vi "X-CAN_Connection_No_Stream_Connection.vi"() -> ()   [LabVIEW 2015]
uses:
  <vilib>/Stratom, Inc/X-CAN for myRIO (API)/X-CAN Class/Type Definitions/CAN_Speed.ctl
  <vilib>/Stratom, Inc/X-Modules for myRIO/Type Defs/MXPChannel.ctl
  <vilib>/Platform/TimedLoop/XDataNode/timing_clust.ctl
  <vilib>/Platform/TimedLoop/XDataNode/nitl_modes.ctl
  <vilib>/Platform/TimedLoop/XDataNode/wakeup.ctl
  <vilib>/platform/TimedLoop/XDataNode/XDataNode.xnode
  <vilib>/Stratom, Inc/X-CAN for myRIO (API)/X-CAN Class/X-CAN.lvclass
  <vilib>/Platform/TimedLoop/XDataNode/XDNodeRunTimeDep.lvlib
panel:
  out "Motor positions (degree)":T1(array[cluster]) {"Error Code (bits)" format="%b"}
  in  "Stop Button":bool
  in  "Enable Joint":bool[](array[boolean])
  in  "Reset?":bool
  in  "Desired position (degrees)":i32[](array[numeric])
  # "Base"
  # "Shoulder"
  # "Elbow"
  # "Wrist"
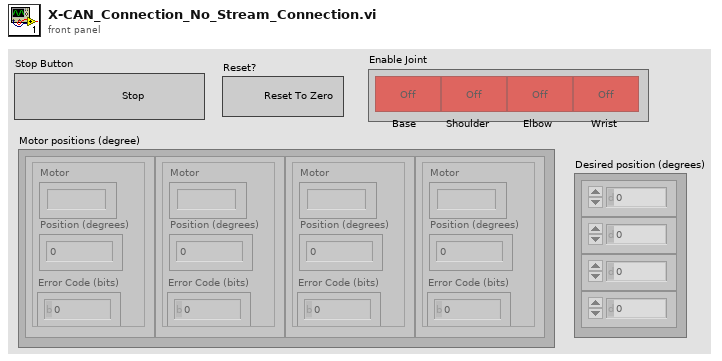
[diagram p1: front panel]
types:
  T1 = cluster{"Position (degrees)":i32, "Error Code (bits)":u8, "Motor":string}[]
  T2 = typedef "MXPChannel.ctl" = enum16{"A/MXP", "B/MXP"}
  T3 = typedef "X-CAN.lvclass/CAN_Speed.ctl" = u8
  T4 = cluster{"ID":u8, "Position":u16, "Error Code":u8}[]
  T5 = typedef "XDNodeRunTimeDep.lvlib/timing_clust.ctl" = cluster{"Expected End [f-1]":u64, "Actual End [f-1]":u64, "Finished Late? [f-1]":bool, "Expected End [i-1]":u64, "Actual End [i-1]":u64, "Finished Late? [i-1]":bool, "Expected Start [i]":u64, "Actual Start [i]":u64, "Expected Start [f]":u64, "Actual Start [f]":u64, "Source Name":string, "Structure Name":string, "Period":i64, "Deadline":i64, "Offset":i64, "Start":i64, "Priority":i32, "Timeout":i32, "Mode":T6, "Wakeup Reason":T7, "Error":errorcluster, "Source Type":string, "Secondary Source Type":string, "Global End Time":u64, "Global Start Time":u64, "Frame Duration":u64, "Iteration Duration":u64, "Assigned CPU":i32, "I/O Scan Engine Mode":u32}
  T6 = typedef "XDNodeRunTimeDep.lvlib/nitl_modes.ctl" = enum32{"No Change", "Process missed periods, maintain original phase", "Discard missed periods, maintain original phase", "Process missed periods, ignore original phase", "Discard missed periods, ignore original phase"}
  T7 = typedef "XDNodeRunTimeDep.lvlib/wakeup.ctl" = enum32{"Normal", "Aborted", "Asynchronous wakeup", "Timing source error", "Timed loop error", "Timeout"}
  T8 = cluster{"ID":u8, "Position":u16, "Error Code":u8}
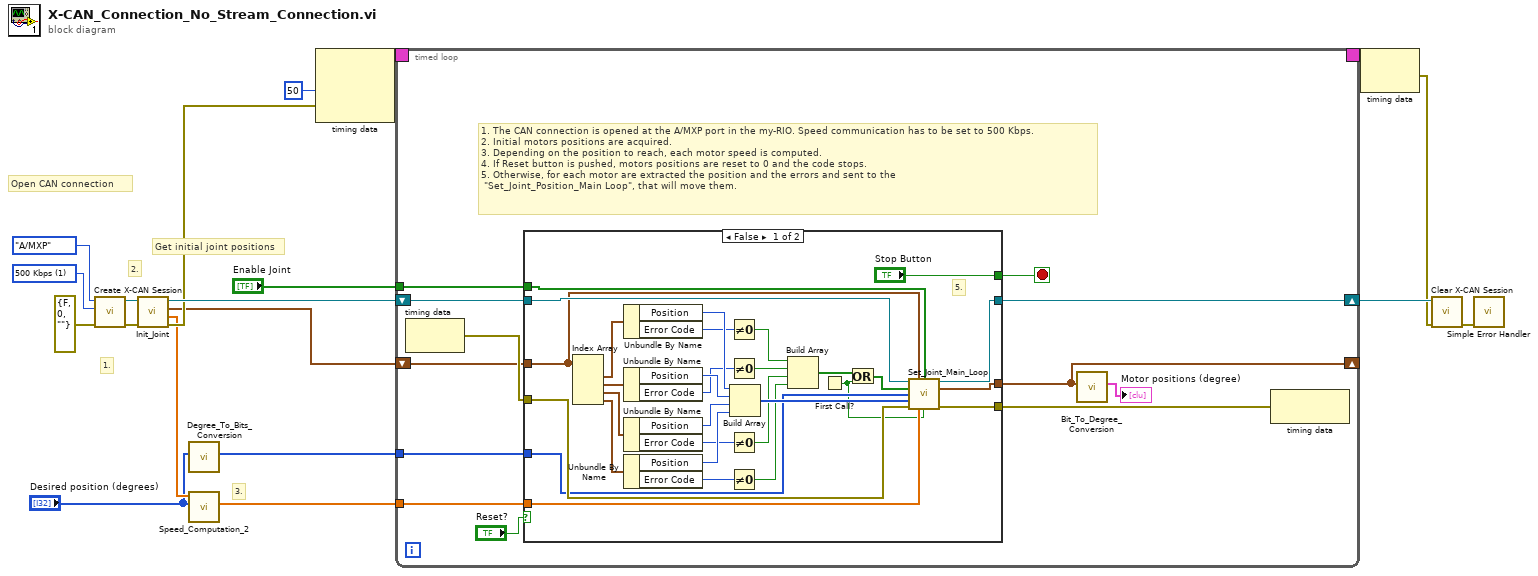
[diagram p0: block diagram]
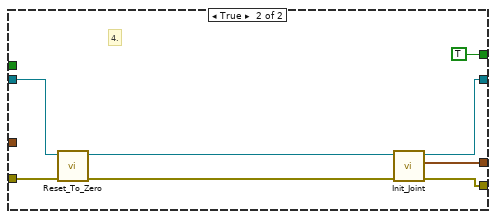
[diagram p2: hidden frame]
diagram:
  w18 = T3 1 items=["125 Kbps"=7, "250 Kbps"=3, "500 Kbps"=1, "1000 Kbps"=0, "95.238 Kbps"=6] ("CAN Speed [Kbps]")
  # "3."
  # "2."
  # "1."
  # "Get initial joint positions"
  # "Open CAN connection"
  n1 = call <vilib>:"Create X-CAN Session.vi"("error in (no error)"=errorcluster {"status"=FALSE, "code"=0, "source"=""}, "CAN Speed [Kbps]"=w18, "MXP Channel"=MXPChannel."A/MXP") -> ("error out"=w9:errorcluster, "X-CAN Session out"=w10:refnum<class "X-CAN.lvclass">)  [unwired: 7 in]
  n2 = call "Init_Joint.vi"("error in"=w9, "X-CAN Session in"=w10) -> ("error out"=w7:errorcluster, "Initial position"=w5:dbl[], "Init Position"=w6:T4, "X-CAN Session out"=w8:refnum<class "X-CAN.lvclass">)  [unwired: 5 in]
  n3 = call "Degree_To_Bits_Conversion.vi"("Degree"="Desired position (degrees)") -> ("Bit positions"=w1:u16[])  [unwired: 10 in]
  n4 = call "Speed_Computation_2.vi"("Desired position"="Desired position (degrees)", "Current position"=w5) -> ("Speed"=w4:dbl[])  [unwired: 9 in]
  n5 = node-c288(i64 50 ("Period"), w7) -> (w16:T5)  [unwired: 1 in]
  n6 = timed-loop {
    timing: w16 -> [_]
    timing-out: [_] -> w15
    shift-right: [w28] -> w13
    shift-left: w8 -> [w31]
    shift-right: [w21] -> _
    shift-left: w6 -> [w27]
    tunnel: w4 -> [w26]
    tunnel: w1 -> [w25]
    tunnel: "Enable Joint" -> [w22]
    stop <- w23 stop-if-true
    # "1. The CAN connection is opened at the A/MXP port in the my-RIO. Speed communication has to be set to 500 Kbps.\n2. Initial motors positions are acquired.\n3. Depending on the position to reach, each motor speed is computed.\n4. If Reset button is pushed, motors positions are reset to 0 and the code stops.\n5. Otherwise, for each motor are extracted the position and the errors and sent to the\n \"Set_Joint_Position_Main Loop\", that will move them."
    n7 = node-c288() -> (w30:errorcluster)  [unwired: 1 in]
    n8 = case shown="False" "Reset?" {
      tunnel: w31 -> [w61 w69]
      tunnel: w30 -> [w60 w68]
      tunnel: [w59 w66] -> w29
      tunnel: [w58 w63] -> w28
      tunnel: [w57 w62] -> w21
      tunnel: w27 -> [w56 _]
      tunnel: w26 -> [w36 _]
      tunnel: w25 -> [w34 _]
      tunnel: ["Stop Button" TRUE ("stop")] -> w23
      tunnel: w22 -> [w35 _]
      frame False {
        # "5."
        n9 = Index Array(array=w56) -> (element #1=w55:T8, element #2=w54:T8, element #3=w53:T8, element #4=w52:T8)  [unwired: 4 in]
        n10 = Unbundle By Name(w55) -> ("Position"=w51:u16, "Error Code"=w46:u8)
        n11 = Unbundle By Name(w54) -> ("Position"=w50:u16, "Error Code"=w44:u8)
        n12 = Unbundle By Name(w53) -> ("Position"=w49:u16, "Error Code"=w42:u8)
        n13 = Unbundle By Name(w52) -> ("Position"=w48:u16, "Error Code"=w40:u8)
        n14 = Not Equal To 0?(x=w46) -> (x != 0?=w45:bool)
        n15 = Not Equal To 0?(x=w44) -> (x != 0?=w43:bool)
        n16 = Not Equal To 0?(x=w42) -> (x != 0?=w41:bool)
        n17 = Not Equal To 0?(x=w40) -> (x != 0?=w39:bool)
        n18 = Build Array(w51, w50, w49, w48) -> (w47:u16[])
        n19 = Build Array(w45, w43, w41, w39) -> (w38:bool[])
        n20 = First Call?() -> (First Call?: T/F=w32:bool)
        n21 = Or(x=w38, y=w32) -> (x .or. y?=w37:bool[])
        n22 = call "Set_Joint_Main_Loop.vi"("X-CAN in"=w61, "Actual position"=w56, "Motor enabled?"=w35, "Reset?"=w37, "Desired position"=w34, "Current position"=w47, "error in (no error)"=w60, "Speed"=w36, "Reset speed?"=w32) -> ("X-CAN out"=w58:refnum<class "X-CAN.lvclass">, "New position"=w57:T4, "error out"=w59:errorcluster)  [unwired: 4 in]
      }
      frame True {
        # "4."
        n23 = call "Reset_To_Zero.vi"("error in"=w68, "X-CAN Session in"=w69) -> ("error out"=w65:errorcluster, "X-CAN Session out"=w64:refnum<class "X-CAN.lvclass">)  [unwired: 8 in]
        n24 = call "Init_Joint.vi"("error in"=w65, "X-CAN Session in"=w64) -> ("error out"=w66:errorcluster, "Init Position"=w62:T4, "X-CAN Session out"=w63:refnum<class "X-CAN.lvclass">)  [unwired: 5 in, 1 out]
      }
    }
    n25 = call "Bit_To_Degree_Conversion.vi"("Actual joints positions"=w21) -> ("Motor positions (degree)"=→"Motor positions (degree)":T1)  [unwired: 10 in]
    n26 = node-c288(w29) -> ()  [unwired: 1 out]
  }
  n27 = node-c288(w15) -> (w11:errorcluster)
  n28 = call <vilib>:"Clear X-CAN Session.vi"("error in (no error)"=w11, "X-CAN Session in"=w13) -> ("error out"=w12:errorcluster)  [unwired: 9 in]
  n29 = call <vilib>:"Simple Error Handler.vi"("error in (no error)"=w12) -> ()  [unwired: 4 in, 5 out]
